vi "SVPO Single Block Integration (1 Ch DBL Array).vi"(9 "known condition":T1={"condition type"=enum."Initial Value", "known value"=nan}, 10 "sampling rate [Hz]":dbl=1.0, 11 "scaled signal [EU]":dbl[](array[numeric])) -> (3 "integrated signal [EU*s]":dbl[](array[numeric]))   [LabVIEW 2017, in "SoundVib_Integration.lvlib"]
doc: "Converts acceleration to velocity or velocity to displacement using a time-domain waveform as the input. Wire data to the <B>scaled signal [EU]</B> input to determine the polymorphic instance to use or manually select the instance. This VI performs Single Integration only. You can pass the integrated signal [EU*s] output to the scaled signal [EU] input of second call to this VI to perform double integration."
uses:
  <vilib>/addons/Sound and Vibration/svt_Integration/SoundVib_Integration.lvlib
  <vilib>/addons/_NISVFA/_Shared subVIs/Controls/svc_Integration Known Condition.ctl
  <vilib>/Analysis/2dsp.llb/Integral Method.ctl
  <vilib>/Analysis/baseanly.llb/Mean (DBL).vi
  <vilib>/Analysis/NI_AALPro.lvlib
  <vilib>/Analysis/NI_AALBase.lvlib
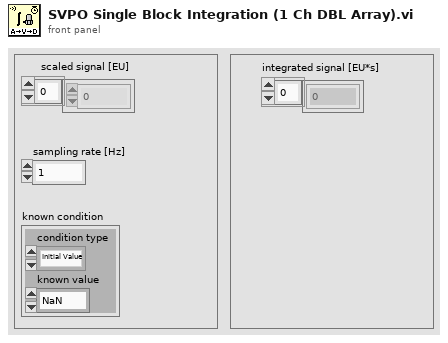
[diagram p1: front panel]
types:
  T1 = typedef "svc_Integration Known Condition.ctl" = cluster{"condition type":enum16{"Initial Value", "Mean Value", "Final Value"}, "known value":dbl}
  T2 = typedef "NI_AALPro.lvlib/Integral Method.ctl" = i32
  T3 = enum16{"Initial Value", "Mean Value", "Final Value"}
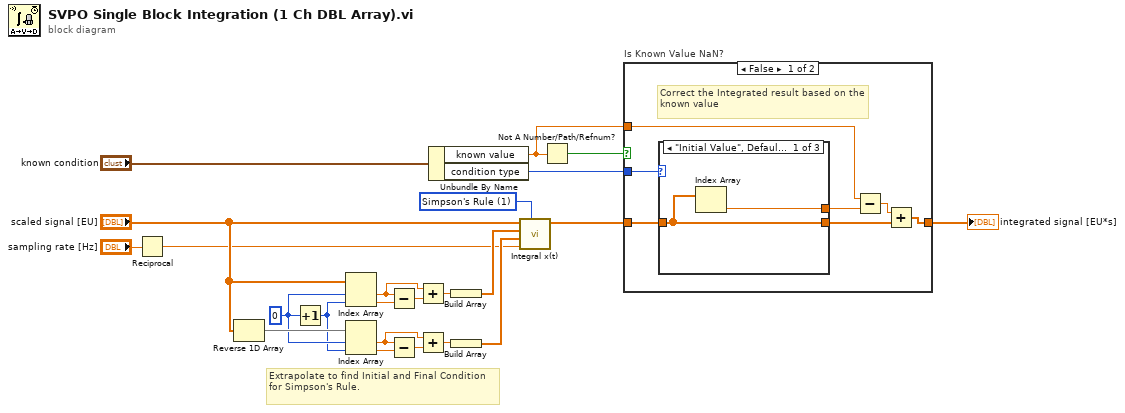
[diagram p0: block diagram]
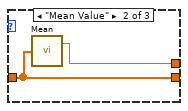
[diagram p2: hidden frame]
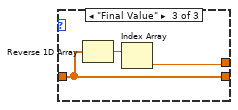
[diagram p3: hidden frame]
diagram:
  w10 = 0
  w22 = T2 1 items=["Trapezoidal Rule", "Simpson's Rule", "Simpson's 3/8 Rule", "Bode Rule"] ("integration method")
  # "Extrapolate to find Initial and Final Condition for Simpson's Rule."
  n1 = Reciprocal(x="sampling rate [Hz]") -> (1/x=w14:dbl)
  n2 = Reverse 1D Array(array="scaled signal [EU]") -> (reversed array=w12:dbl[])
  n3 = Increment(x=w10) -> (x+1=w9:i32)
  n4 = Index Array(array="scaled signal [EU]", index #1=w10, index #2=w9) -> (element #1=w7:dbl, element #2=w8:dbl)
  n5 = Index Array(array=w12, index #1=w10, index #2=w9) -> (element #1=w2:dbl, element #2=w3:dbl)
  n6 = Subtract(x=w7, y=w8) -> (x-y=w6:dbl)
  n7 = Subtract(x=w2, y=w3) -> (x-y=w5:dbl)
  n8 = Add(x=w7, y=w6) -> (x+y=w11:dbl)
  n9 = Add(x=w2, y=w5) -> (x+y=w4:dbl)
  n10 = Unbundle By Name("known condition") -> ("known value"=w17:dbl, "condition type"=w1:T3)
  n11 = Build Array(w11) -> (w20:dbl[])
  n12 = Build Array(w4) -> (w21:dbl[])
  n13 = call <vilib>:"Integral x(t).vi"("integration method"=w22, "dt"=w14, "Final Condition"=w21, "Initial Condition"=w20, "X"="scaled signal [EU]") -> ("Integral X"=w18:dbl[])  [unwired: 5 in, 1 out]
  n14 = Not A Number/Path/Refnum?(number/path/refnum=w17) -> (NaN/Path/Refnum?=w19:bool)
  n15 = case "Is Known Value NaN?" shown="False" w19 {
    tunnel: [w27 w38] -> w13
    tunnel: w18 -> [w30 w38]
    tunnel: w17 -> [w26 _]
    tunnel: w1 -> [w24 _]
    frame False {
      # "Correct the Integrated result based on the known value"
      n16 = case shown="\"Initial Value\", Default" w24 {
        tunnel: w30 -> [w31 w34 w36]
        tunnel: [w31 w34 w36] -> w28
        tunnel: [w32 w33 w35] -> w25
        frame "Initial Value", Default {
          n17 = Index Array(array=w31) -> (element=w32:dbl)  [unwired: 1 in]
        }
        frame "Mean Value" {
          n18 = call-poly <vilib>:"Mean.vi"("X"=w34) -> ("mean"=w33:dbl)  [unwired: 1 out]
        }
        frame "Final Value" {
          n19 = Reverse 1D Array(array=w36) -> (reversed array=w37:dbl[])
          n20 = Index Array(array=w37) -> (element=w35:dbl)  [unwired: 1 in]
        }
      }
      n21 = Subtract(x=w26, y=w25) -> (x-y=w29:dbl)
      n22 = Add(x=w29, y=w28) -> (x+y=w27:dbl[])
    }
    frame True {
      # "No operation when Known Value is NaN. When Known Value is NaN we assume an initial value of zero"
    }
  }
  "integrated signal [EU*s]" <- w13
